vi "Initialize.vi"(6 "Actor Name":string, 7 "Host Name":string, 8 "error in (no error)":errorcluster, 11 "Message Broker Interface":refnum<class "Message Broker Interface.lvclass">) -> (0 "error out":errorcluster, 3 "Car Position Simulator out":refnum<class "Car Position Simulator.lvclass">)   [LabVIEW 2016, in "CLD Exam - Car Wash.lvlib" / "Car Position Simulator.lvclass"]
uses:
  Car Position Simulator.lvclass
  Mediator/Classes/Message Broker Interface/Message Broker Interface.lvclass
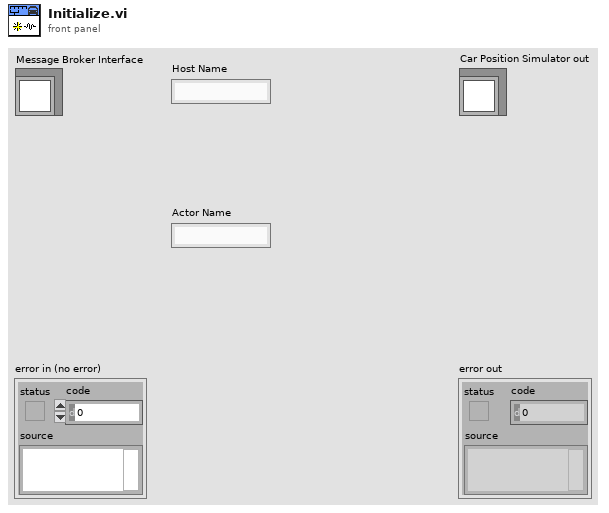
[diagram p1: front panel]
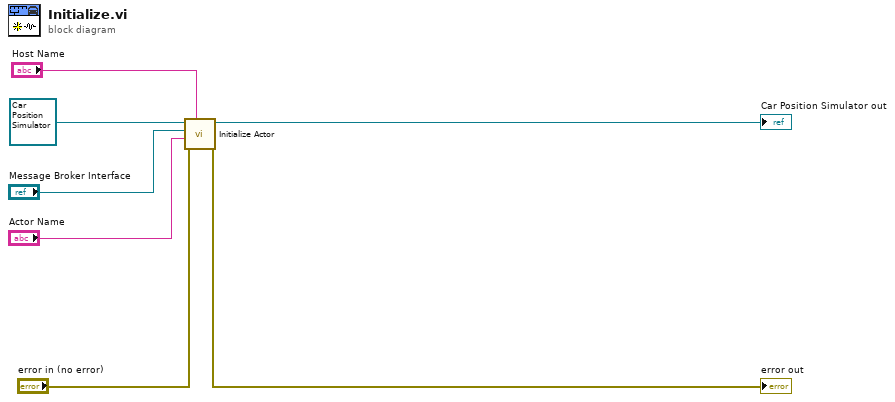
[diagram p0: block diagram]
diagram:
  n1 = call-dynamic "Initialize Actor.vi"("Host Name"="Host Name", "error in (no error)"="error in (no error)", "Actor Name"="Actor Name", "Message Broker Interface"="Message Broker Interface", "Car Position Simulator in"=refnum<class "Car Position Simulator.lvclass"> refnum) -> ("error out"=→"error out":errorcluster, "Car Position Simulator out"=→"Car Position Simulator out":refnum<class "Car Position Simulator.lvclass">)  [unwired: 5 in]
